vi "test.vi"() -> ()   [LabVIEW 2010, in "GenericDigitalOut.lvclass"]
uses:
  GenericDigitalOut.lvclass
  common/classes/GenericComponent/GenericComponent/GenericComponent.lvclass
panel:
  out "high?":bool
  in  "create button":bool
  in  "stop":bool
  in  "toggle button":bool
  in  "configure button":bool
  # "Test suite for DigitalOut components"
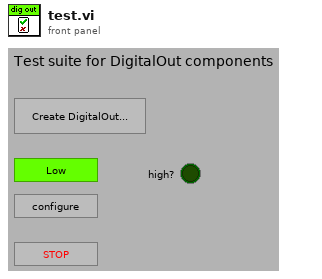
[diagram p1: front panel]
types:
  T1 = typedef "XComponentSpecification.xctl/data.ctl" = cluster{"class path":string, "configuration":string, "label":string, "settings name":string}
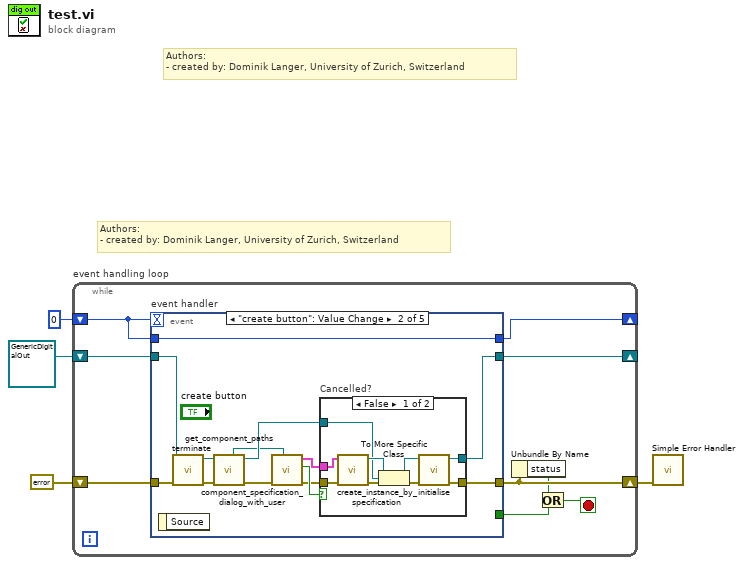
[diagram p0: block diagram]
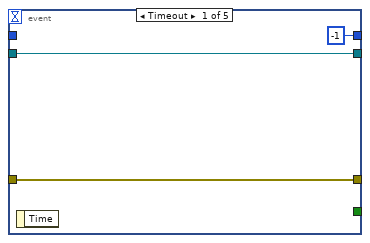
[diagram p2: hidden frame]
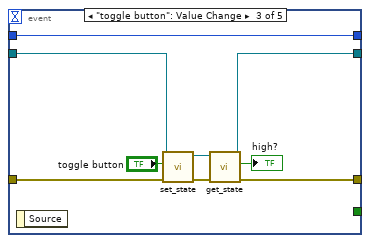
[diagram p4: hidden frame]
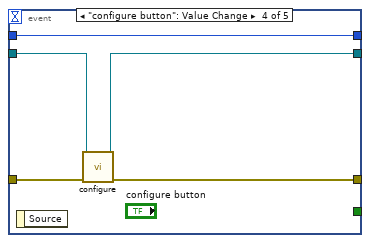
[diagram p5: hidden frame]
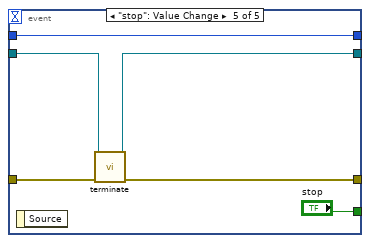
[diagram p6: hidden frame]
diagram:
  # "Authors: \n- created by: Dominik Langer, University of Zurich, Switzerland"
  # "Authors: \n- created by: Dominik Langer, University of Zurich, Switzerland"
  n1 = while "event handling loop" {
    shift-right: [w8] -> w2
    shift-left: errorcluster {"status"=FALSE, "code"=0, "source"=""} ("error out") -> [w13]
    shift-right: [w9] -> _
    shift-left: refnum<class "GenericDigitalOut.lvclass"> refnum ("GenericDigitalOut.lvclass") -> [w12]
    shift-right: [w10] -> _
    shift-left: 0 -> [w11]
    stop <- w6 stop-if-true
    n2 = event "event handler" shown="[1] \"create button\": Value Change" {
      selector: _ -> [_ _ _ _ _]
      dyn-events: _ -> [_ _ _ _ _]
      timeout: w11 -> [_ _ _ _ _]
      tunnel: w13 -> [w14 w28 w48 w53 w59]
      tunnel: [w14 w18 w44 w52 w58] -> w8
      tunnel: w12 -> [w15 w27 w47 w51 w57]
      tunnel: w11 -> [_ w29 w49 w54 w60]
      tunnel: [-1 w29 w49 w54 w60] -> w10
      tunnel: [w15 w19 w42 w50 w56] -> w9
      tunnel: [_ _ _ _ "stop"] -> w5
      event Timeout {
        n3 = event-data() -> ()  [unwired: 2 out]
      }
      event "create button": Value Change {
        n4 = event-data() -> ()  [unwired: 2 out]
        n5 = call-dynamic "terminate.vi"("error in (no error)"=w28, "GenericPlugin in"=w27) -> ("error out"=w20:errorcluster, "GenericPlugin out"=w17:refnum<class "GenericDigitalOut.lvclass">)  [unwired: 8 out]
        n6 = call-dynamic "get_component_paths.vi"("error in (no error)"=w20, "GenericComponent in"=w17) -> ("error out"=w21:errorcluster, "GenericComponent out"=w24:refnum<class "GenericDigitalOut.lvclass">, "component type directory"=w23:path)  [unwired: 4 in, 3 out]
        n7 = call "component_specification_dialog_with_user.vi"("start path"=w23, "error in (no error)"=w21) -> ("error out"=w22:errorcluster, "cancelled?"=w25:bool, "component specification out"=w26:T1)  [unwired: 7 in]
        n8 = case "Cancelled?" shown="False" w25 {
          tunnel: [w31 w40] -> w18
          tunnel: w22 -> [w36 w40]
          tunnel: w24 -> [w35 w39]
          tunnel: w26 -> [w34 _]
          tunnel: [w30 w39] -> w19
          frame False {
            n9 = call "create_instance_by_specification.vi"("error in (no error)"=w36, "component specification"=w34) -> ("error out"=w38:errorcluster, "GenericPlugin out"=w37:refnum<class "GenericComponent.lvclass">)  [unwired: 7 in, 1 out]
            n10 = To More Specific Class(target class=w35, reference=w37, error in=w38) -> (specific class reference=w32:refnum<class "GenericDigitalOut.lvclass">, error out=w33:errorcluster)
            n11 = call-dynamic "initialise.vi"("error in (no error)"=w33, "GenericPlugin in"=w32) -> ("error out"=w31:errorcluster, "GenericPlugin out"=w30:refnum<class "GenericDigitalOut.lvclass">)  [unwired: 8 out]
          }
          frame True {
          }
        }
      }
      event "toggle button": Value Change {
        n12 = event-data() -> ()  [unwired: 2 out]
        n13 = call-dynamic "set_state.vi"("error in (no error)"=w48, "state"="toggle button", "GenericDigitalOut in"=w47) -> ("error out"=w45:errorcluster, "GenericDigitalOut out"=w43:refnum<class "GenericDigitalOut.lvclass">)  [unwired: 7 in]
        n14 = call-dynamic "get_state.vi"("error in (no error)"=w45, "GenericDigitalOut in"=w43) -> ("error out"=w44:errorcluster, "state"=→"high?":bool, "GenericDigitalOut out"=w42:refnum<class "GenericDigitalOut.lvclass">)  [unwired: 7 in]
      }
      event "configure button": Value Change {
        n15 = event-data() -> ()  [unwired: 2 out]
        n16 = call-dynamic "configure.vi"("error in (no error)"=w53, "GenericPlugin in"=w51) -> ("error out"=w52:errorcluster, "GenericPlugin out"=w50:refnum<class "GenericDigitalOut.lvclass">)  [unwired: 8 out]
      }
      event "stop": Value Change {
        n17 = event-data() -> ()  [unwired: 2 out]
        n18 = call-dynamic "terminate.vi"("error in (no error)"=w59, "GenericPlugin in"=w57) -> ("error out"=w58:errorcluster, "GenericPlugin out"=w56:refnum<class "GenericDigitalOut.lvclass">)  [unwired: 8 out]
      }
    }
    n19 = Unbundle By Name(w8) -> ("status"=w7:bool)
    n20 = Or(x=w7, y=w5) -> (x .or. y?=w6:bool)
  }
  n21 = call <vilib>:"Simple Error Handler.vi"("error in (no error)"=w2) -> ()  [unwired: 1 in, 8 out]
